vi "Peak detector.vi"(11 "Filtered X":dbl[](array[numeric])) -> (3 "Numeric":i32)   [LabVIEW 2018]
uses:
  <vilib>/Analysis/NI_AALPro.lvlib
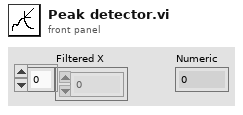
[diagram p1: front panel]
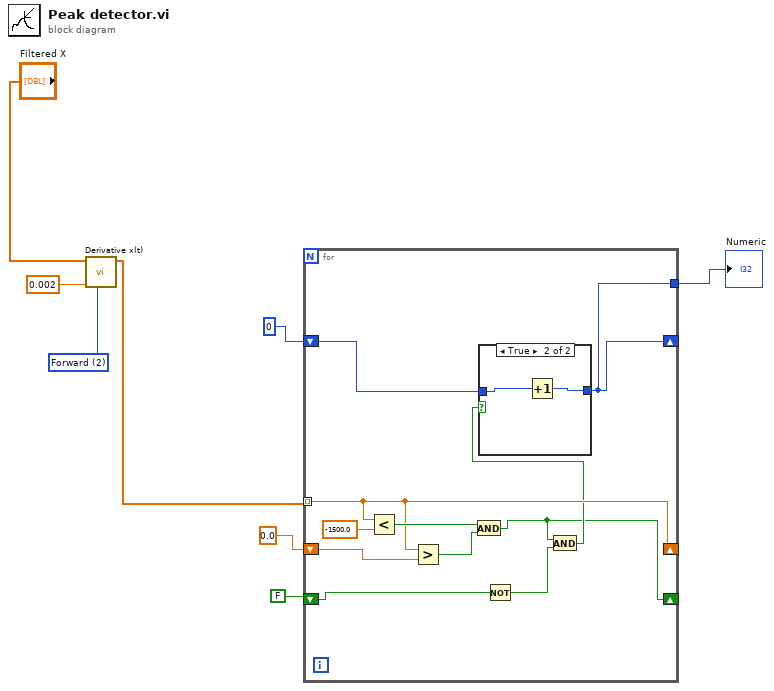
[diagram p0: block diagram]
diagram:
  w2 = u16 2 items=["2nd Order Central", "4th Order Central", "Forward", "Backward"] ("method")
  n1 = call <vilib>:"Derivative x(t).vi"("method"=w2, "dt"=0.002, "X"="Filtered X") -> ("dX/dt"=w5:dbl[])  [unwired: 7 in, 1 out]
  n2 = for {
    shift-right: [w18] -> _
    shift-left: 0 -> [w19]
    tunnel: w5 -> [w15] mode=indexing
    shift-right: [w15] -> _
    shift-left: 0.0 -> [w14]
    tunnel: [w18] -> w8
    shift-right: [w9] -> _
    shift-left: FALSE -> [w12]
    n3 = Less?(x=w15, y=-1500.0) -> (x < y?=w16:bool)
    n4 = Greater?(x=w15, y=w14) -> (0:w13:bool)
    n5 = And(x=w16, y=w13) -> (x .and. y?=w9:bool)
    n6 = Not(x=w12) -> (.not. x?=w11:bool)
    n7 = And(x=w9, y=w11) -> (x .and. y?=w10:bool)
    n8 = case shown="True" w10 {
      tunnel: w19 -> [w20 w22]
      tunnel: [w20 w21] -> w18
      frame False {
      }
      frame True {
        n9 = Increment(x=w22) -> (x+1=w21:i32)
      }
    }
  }
  "Numeric" <- w8
